vi "Write Cal Standard Port.vi"(8 "error in (no error)":errorcluster, 10 "Cal Standard Port":string, 11 "Vector Path in":refnum<class "Vector Abstract Path.lvclass">) -> (0 "error out":errorcluster, 3 "Vector Path out":refnum<class "Vector Abstract Path.lvclass">)   [LabVIEW 2023, in "RFFixtureCharact.Public.lvlib" / "Vector Abstract Path.lvclass"]
uses:
  Vector Abstract Path.lvclass
  Vector Abstract Path.lvclass/Vector Abstract Path.ctl
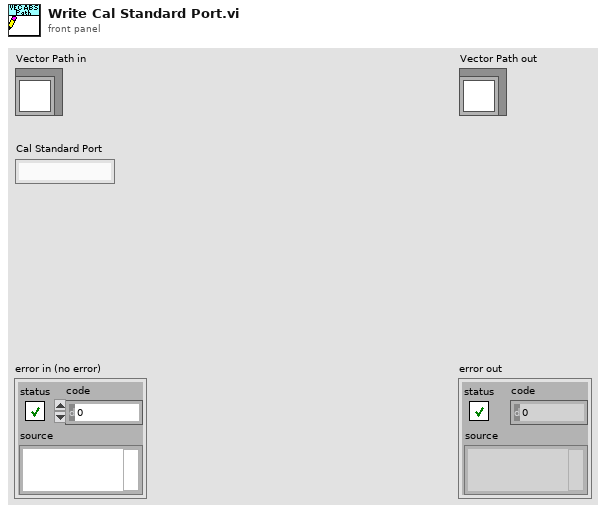
[diagram p1: front panel]
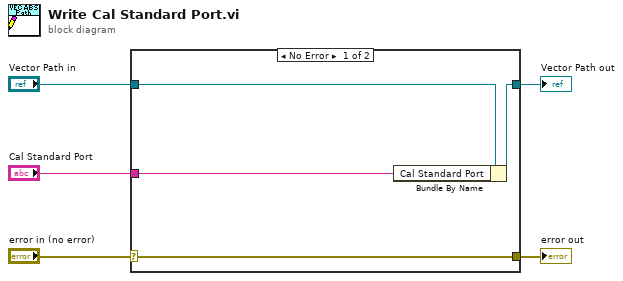
[diagram p0: block diagram]
diagram:
  n1 = case shown="No Error" "error in (no error)" {
    selector: "error in (no error)" -> [w9 w10]
    tunnel: [w9 w10] -> w4
    tunnel: [w7 w11] -> w2
    tunnel: "Vector Path in" -> [w8 w11]
    tunnel: "Cal Standard Port" -> [w6 _]
    frame No Error {
      n2 = Bundle By Name(cluster=w8, "Cal Standard Port"=w6) -> (w7:refnum<class "Vector Abstract Path.lvclass">)
    }
    frame Error {
    }
  }
  "error out" <- w4
  "Vector Path out" <- w2
